vi "STATUS VACON.vi"() -> ()   [LabVIEW 2019]
panel:
  out "STATUS VACON":T1
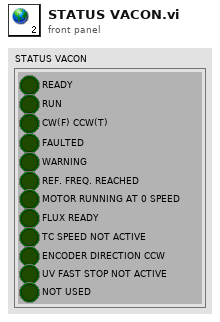
[diagram p1: front panel]
types:
  T1 = cluster{"READY":bool, "RUN":bool, "CW(F) CCW(T)":bool, "FAULTED":bool, "WARNING":bool, "REF. FREQ. REACHED":bool, "MOTOR RUNNING AT 0 SPEED":bool, "FLUX READY":bool, "TC SPEED NOT ACTIVE":bool, "ENCODER DIRECTION CCW":bool, "UV FAST STOP NOT ACTIVE":bool, "NOT USED":bool}
diagram:
